vi "Problem 7.vi"() -> ()   [LabVIEW 2025]
uses:
  <vilib>/gmath/NI_AAL_MathFunc.lvlib
panel:
  out "Time To Execute (ms)":dbl
  out "10001st Prime Number":i32
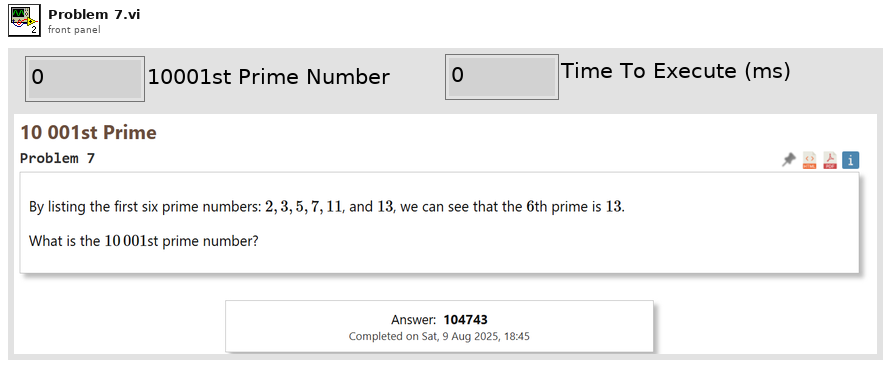
[diagram p1: front panel]
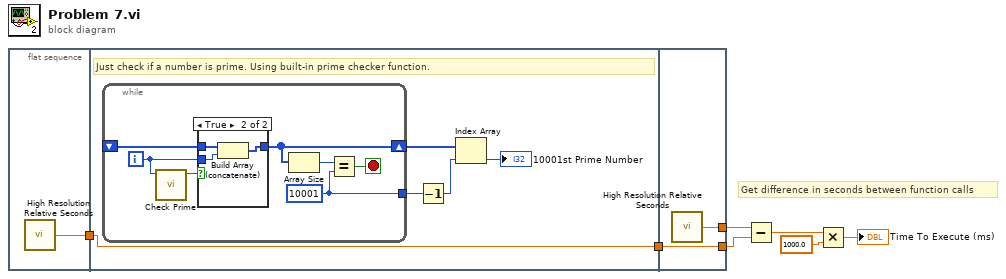
[diagram p0: block diagram]
diagram:
  # "Get difference in seconds between function calls"
  n1 = flat-sequence {
    tunnel: [w8] -> w7
    tunnel: w7 -> [w9]
    tunnel: [w9] -> w6
    tunnel: w6 -> [w26]
    tunnel: [w26] -> w5
    tunnel: [w25] -> w4
    frame #0 {
      n2 = call <vilib>:"High Resolution Relative Seconds.vi"() -> ("relative seconds"=w8:dbl)
    }
    frame #1 {
      # "Just check if a number is prime. Using built-in prime checker function."
      n3 = while {
        shift-right: [w16] -> w13
        shift-left: _ -> [w15]
        tunnel: [w14] -> w11
        i -> [w17]
        stop <- w19 stop-if-true
        w14 = 10001 ("y")
        n4 = call <vilib>:"Check Prime.vi"("n"=w17) -> ("prime?"=w18:bool)  [unwired: 10 in]
        n5 = case shown="True" w18 {
          tunnel: w17 -> [_ w22]
          tunnel: [w21 w24] -> w16
          tunnel: w15 -> [w21 w23]
          frame False {
          }
          frame True {
            n6 = Build Array (concatenate)(w23, w22) -> (w24:i32[])
          }
        }
        n7 = Array Size(array=w16) -> (size(s)=w20:i32)
        n8 = Equal?(x=w20, y=w14) -> (x = y?=w19:bool)
      }
      n9 = Decrement(x=w11) -> (x-1=w10:i32)
      n10 = Index Array(array=w13, index=w10) -> (element=→"10001st Prime Number":i32)
    }
    frame #2 {
      n11 = call <vilib>:"High Resolution Relative Seconds.vi"() -> ("relative seconds"=w25:dbl)
    }
  }
  n12 = Subtract(x=w4, y=w5) -> (x-y=w3:dbl)
  n13 = Multiply(x=w3, y=1000.0) -> (x*y=→"Time To Execute (ms)":dbl)
